vi "Power_Supply Get Attributes.vi"(8 "error in (no error)":errorcluster, 11 "PXIe-4130 in":refnum<class "PXIe-4130.lvclass">) -> (0 "error out":errorcluster, 2 "Class Attributes":T1, 3 "PXIe-4130 out":refnum<class "PXIe-4130.lvclass">)   [LabVIEW 2018, in "PXIe-4130.lvclass"]
uses:
  PXIe-4130.lvclass
  Controls/Class Attributes Cluster.ctl
  PXIe-4130.lvclass/PXIe-4130.ctl
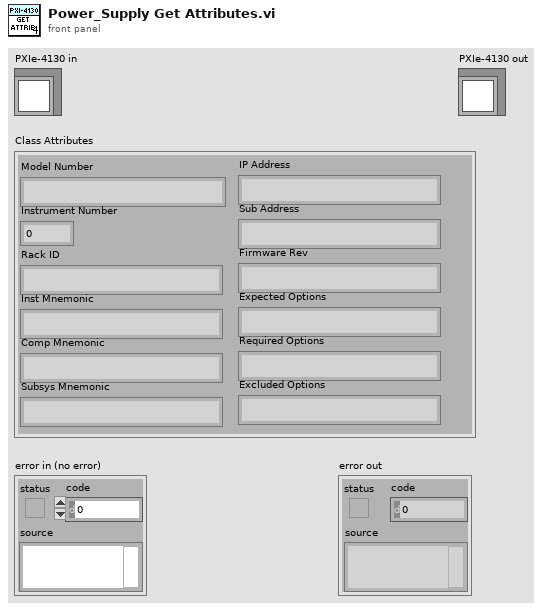
[diagram p1: front panel]
types:
  T1 = typedef "Class Attributes Cluster.ctl" = cluster{"Model Number":string, "Instrument Number":u8, "Rack ID":string, "Inst Mnemonic":string, "Comp Mnemonic":string, "Subsys Mnemonic":string, "IP Address":string, "Sub Address":string, "Firmware Rev":string, "Expected Options":string, "Required Options":string, "Excluded Options":string}
  T2 = typedef "Class Instrument Info.ctl" = string[]
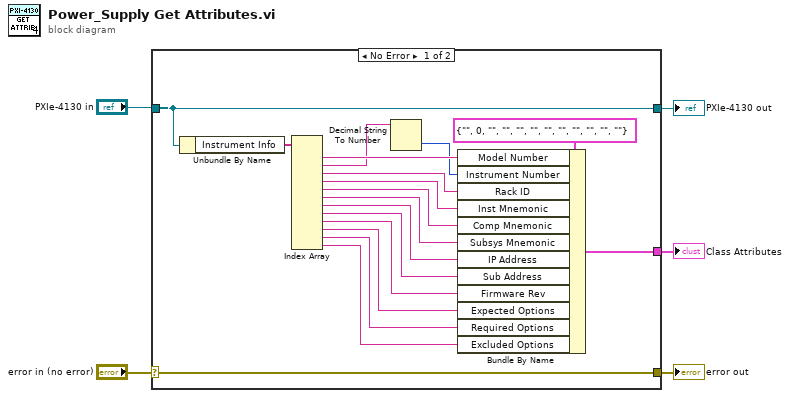
[diagram p0: block diagram]
diagram:
  n1 = case shown="No Error" "error in (no error)" {
    selector: "error in (no error)" -> [w23 w25]
    tunnel: [w23 w25] -> w4
    tunnel: [w6 w24] -> w1
    tunnel: "PXIe-4130 in" -> [w6 w24]
    tunnel: [w7 _] -> w3
    frame No Error {
      n2 = Unbundle By Name(w6) -> ("Instrument Info"=w22:T2)
      n3 = Index Array(array=w22) -> (element #1=w20:string, element #2=w19:string, element #3=w17:string, element #4=w16:string, element #5=w15:string, element #6=w14:string, element #7=w13:string, element #8=w12:string, element #9=w11:string, element #10=w10:string, element #11=w9:string, element #12=w8:string)  [unwired: 12 in]
      n4 = Decimal String To Number(string=w19) -> (number=w18:i32)  [unwired: 2 in, 1 out]
      n5 = Bundle By Name(cluster=T1 {"Model Number"="", "Instrument Number"=0, "Rack ID"="", "Inst Mnemonic"="", "Comp Mnemonic"="", "Subsys Mnemonic"="", "IP Address"="", "Sub Address"="", "Firmware Rev"="", "Expected Options"="", "Required Options"="", "Excluded Options"=""} ("Class Attributes"), "Model Number"=w20, "Instrument Number"=w18, "Rack ID"=w17, "Inst Mnemonic"=w16, "Comp Mnemonic"=w15, "Subsys Mnemonic"=w14, "IP Address"=w13, "Sub Address"=w12, "Firmware Rev"=w11, "Expected Options"=w10, "Required Options"=w9, "Excluded Options"=w8) -> (w7:T1)
    }
    frame Error {
    }
  }
  "PXIe-4130 out" <- w1
  "error out" <- w4
  "Class Attributes" <- w3
